vi "add Element to Array.vi"(8 "error in (no error)":errorcluster, 9 "Parcour_element.lvclass":refnum<class "Parcour_element.lvclass">, 11 "parcour_Liste in":refnum<class "parcour_Liste.lvclass">) -> (0 "error out":errorcluster, 3 "parcour_Liste out":refnum<class "parcour_Liste.lvclass">)   [LabVIEW 2019, in "parcour_Liste.lvclass"]
uses:
  parcour_Liste.lvclass
  parcour/Parcour_element.lvclass
  parcour_Liste.lvclass/parcour_Liste.ctl
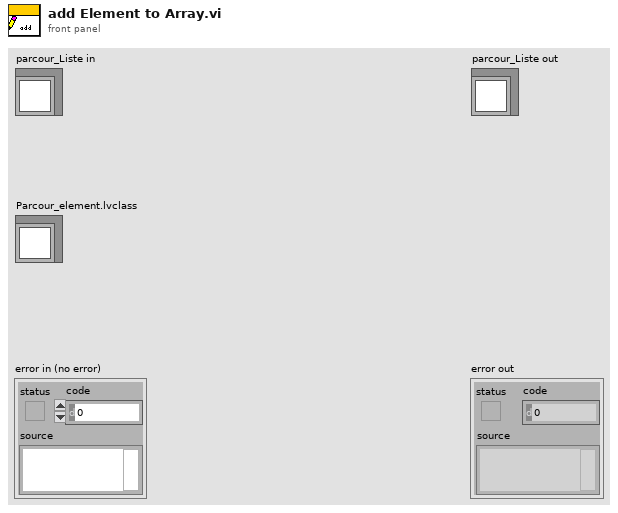
[diagram p1: front panel]
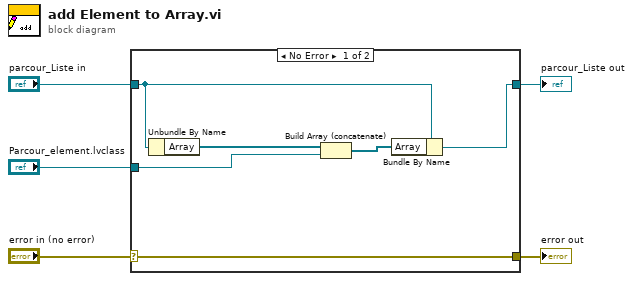
[diagram p0: block diagram]
diagram:
  n1 = case shown="No Error" "error in (no error)" {
    selector: "error in (no error)" -> [w11 w12]
    tunnel: [w11 w12] -> w4
    tunnel: [w10 w13] -> w2
    tunnel: "parcour_Liste in" -> [w9 w13]
    tunnel: "Parcour_element.lvclass" -> [w6 _]
    frame No Error {
      n2 = Unbundle By Name(w9) -> ("Array"=w8:refnum<class "Parcour_element.lvclass">[])
      n3 = Build Array (concatenate)(w8, w6) -> (w7:refnum<class "Parcour_element.lvclass">[])
      n4 = Bundle By Name(cluster=w9, "Array"=w7) -> (w10:refnum<class "parcour_Liste.lvclass">)
    }
    frame Error {
    }
  }
  "error out" <- w4
  "parcour_Liste out" <- w2
